vi "EME 185B LabVIEW.vi"() -> ()   [LabVIEW 2025]
uses:
  <vilib>/Instr/_visa.llb/VISA Configure Serial Port (Instr).vi
  <vilib>/Utility/file.llb/Write Delimited Spreadsheet (string).vi
  <vilib>/Utility/file.llb/Write Delimited Spreadsheet (DBL).vi
panel:
  out "XY Graph":cluster{dbl[], dbl[]}(graph)
  out "VISA resource name out":refnum<visa-resource-name>
  out "Elapsed Time (sec)":dbl
  in  "Seconds per data point":dbl
  in  "stop":bool
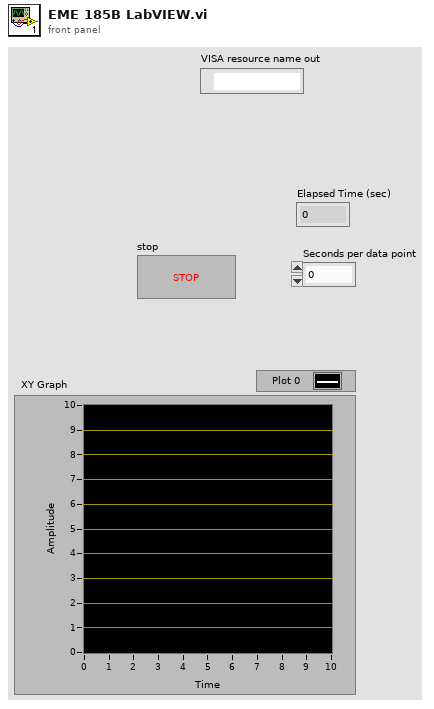
[diagram p1: front panel]
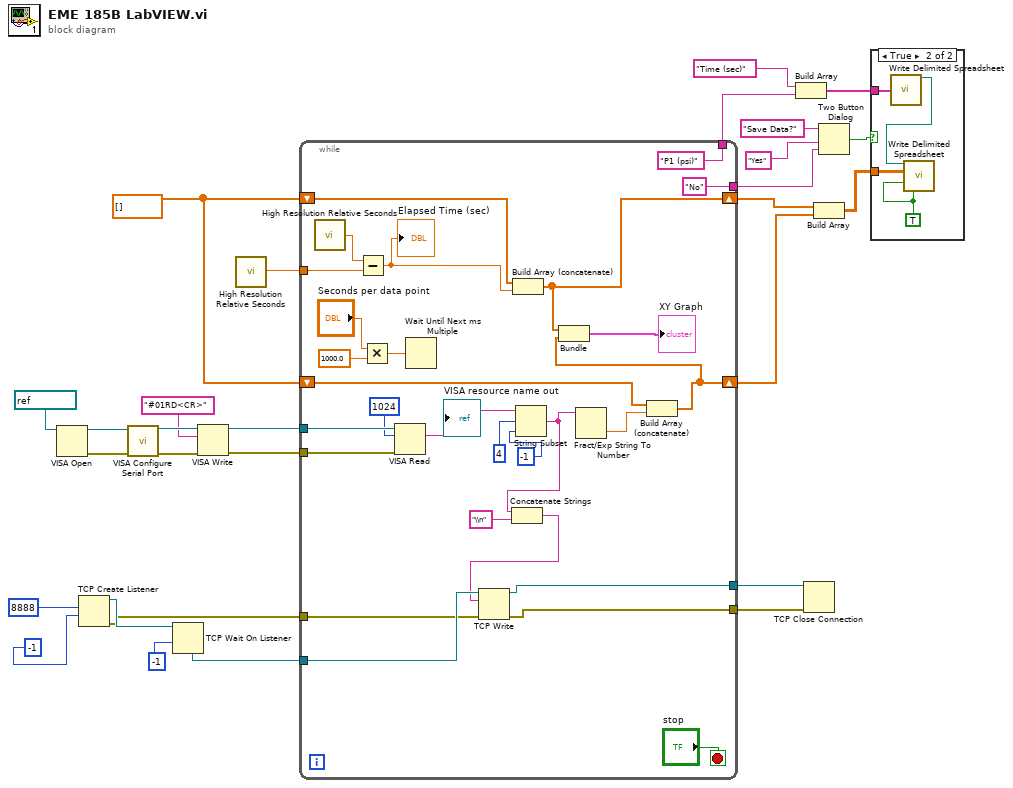
[diagram p0: block diagram]
diagram:
  w17 = dbl[] []
  n1 = VISA Open(VISA resource name=refnum<visa-resource-name> "COM3") -> (VISA resource name=w27:refnum<visa-resource-name>, error out=w26:errorcluster)  [unwired: 4 in]
  n2 = TCP Create Listener(9:-1 ("timeout ms (25000)"), 10:u16 8888 ("port")) -> (0:w3:errorcluster, 3:w4:refnum<k5>)  [unwired: 3 in, 1 out]
  n3 = call-poly "VISA Configure Serial Port"("VISA resource name"=w27, "error in (no error)"=w26) -> ("VISA resource name out"=w25:refnum<visa-resource-name>, "error out"=w5:errorcluster)  [unwired: 12 in]
  n4 = TCP Wait On Listener(9:-1 ("timeout ms (wait forever: -1)"), 11:w4) -> (4:w8:refnum<k5>)  [unwired: 2 in, 4 out]
  n5 = VISA Write(VISA resource name=w25, write buffer="#01RD<CR>", error in (no error)=w5) -> (VISA resource name out=w23:refnum<visa-resource-name>, error out=w22:errorcluster)  [unwired: 1 out]
  n6 = call <vilib>:"High Resolution Relative Seconds.vi"() -> ("relative seconds"=w21:dbl)
  n7 = while {
    tunnel: w23 -> [w56]
    tunnel: w22 -> [w55]
    tunnel: w21 -> [w48]
    shift-right: [w41] -> w20
    shift-left: w17 -> [w46]
    shift-right: [w40] -> w19
    shift-left: w17 -> [w42]
    tunnel: ["P1 (psi)"] -> w14
    tunnel: ["No" ("F button name (\"Cancel\")")] -> w10
    tunnel: w8 -> [w36]
    tunnel: [w32] -> w7
    tunnel: [w31] -> w6
    tunnel: w3 -> [w30]
    stop <- "stop" stop-if-true
    n8 = call <vilib>:"High Resolution Relative Seconds.vi"() -> ("relative seconds"=w49:dbl)
    n9 = Subtract(x=w49, y=w48) -> (x-y=w47:dbl)
    "Elapsed Time (sec)" <- w47
    n10 = Multiply(x="Seconds per data point", y=1000.0) -> (x*y=w52:dbl)
    n11 = VISA Read(VISA resource name=w56, byte count=u32 1024, error in (no error)=w55) -> (read buffer=w29:string)  [unwired: 3 out]
    "VISA resource name out" <- w29
    n12 = Wait Until Next ms Multiple(millisecond multiple=w52) -> ()  [unwired: 1 out]
    n13 = Build Array (concatenate)(w46, w47) -> (w41:dbl[])
    n14 = String Subset(string=w29, offset (0)=4, length (rest)=-1 ("length (rest)")) -> (substring=w35:string)
    n15 = Concatenate Strings(w35, "\\n" ("string")) -> (w33:string)
    n16 = TCP Write(connection ID=w36, data in=w33, error in (no error)=w30) -> (connection ID out=w31:refnum<k5>, error out=w32:errorcluster)  [unwired: 1 in, 1 out]
    n17 = Fract/Exp String To Number(string=w35) -> (number=w43:dbl)  [unwired: 3 in, 1 out]
    n18 = Build Array (concatenate)(w42, w43) -> (w40:dbl[])
    n19 = Bundle(w41, w40) -> (→"XY Graph":cluster{dbl[], dbl[]})  [unwired: 1 in]
  }
  n20 = Build Array("Time (sec)", w14) -> (w15:string[])
  n21 = TCP Close Connection(connection ID=w6, error in (no error)=w7) -> ()  [unwired: 1 in, 2 out]
  n22 = Build Array(w20, w19) -> (w18:dbl[][])
  n23 = Two Button Dialog(message="Save Data?", 1:w10, 2:"Yes" ("T button name (\"OK\")")) -> (T button?=w13:bool)
  n24 = case shown="True" w13 {
    tunnel: w18 -> [_ w60]
    tunnel: w15 -> [_ w59]
    frame False {
    }
    frame True {
      w57 = TRUE ("transpose? (no:F)")
      n25 = call-poly <vilib>:"Write Delimited Spreadsheet.vi"("1D data"=w59) -> ("new file path (Not A Path if cancelled)"=w58:path)  [unwired: 13 in, 1 out]
      n26 = call-poly <vilib>:"Write Delimited Spreadsheet.vi"("file path (dialog if empty)"=w58, "2D data"=w60, "append to file? (new file:F)"=w57, "transpose? (no:F)"=w57) -> ()  [unwired: 10 in, 2 out]
    }
  }
